vi "delay.vi"(8 "error in":errorcluster, 10 "Milliseconds to wait":i32=50, 11 "VISA resource name":refnum<visa-resource-name>) -> (0 "error out":errorcluster, 3 "VISA resource name out":refnum<visa-resource-name> caption="VISA resource name")   [LabVIEW 2014, in "rszvl_rsidr_core.lvlib"]
uses:
  rszvl_rsidr_core.lvlib
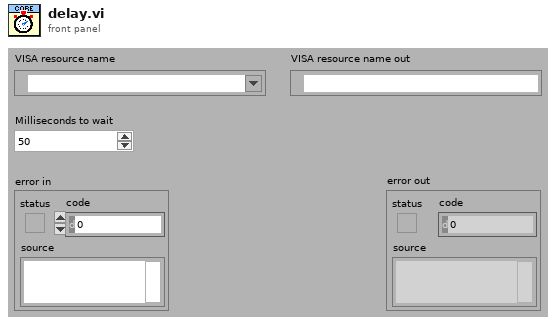
[diagram p1: front panel]
types:
  T1 = typedef "rszvl_rsidr_core.lvlib/type_Session_Data.ctl" = cluster{"Instr type":string, "Instr type for err. msg.":string, "Installed Options":string[], "OPC Timeout":i32, "Query Instrument Status":bool, "Check Range":bool, "Check Options":bool, "Add LF to Write":bool, "Simulate":bool, "Logging":bool, "Logging params":variant, "Interface Type":enum16{"Unknown", "GPIB", "VXI", "GPIB_VXI", "ASRL", "PXI", "TCPIP", "USB", "SOCKET"}, "Fast Sweep":i32, "AdditionalFlags":i32, "WaitBeforeWrite":i32, "WaitBeforeRead":i32, "BinDataChunkSize":i64}
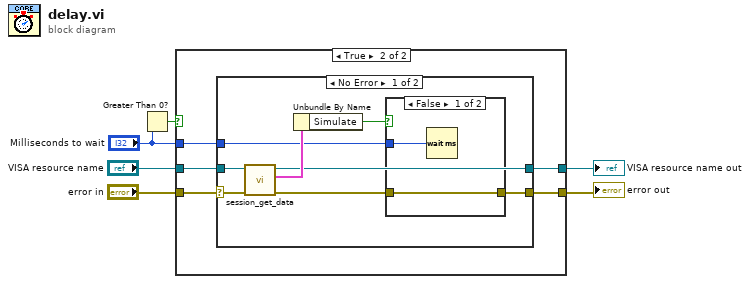
[diagram p0: block diagram]
diagram:
  n1 = Greater Than 0?(x="Milliseconds to wait") -> (x > 0?=w2:bool)
  n2 = case shown="True" w2 {
    tunnel: [w8 w13] -> w6
    tunnel: "VISA resource name" -> [w7 w12]
    tunnel: "error in" -> [w8 w11]
    tunnel: "Milliseconds to wait" -> [_ w10]
    tunnel: [w7 w9] -> w1
    frame False {
    }
    frame True {
      n3 = case shown="No Error" w11 {
        selector: w11 -> [w20 w26]
        tunnel: [w21 w26] -> w13
        tunnel: w12 -> [w19 w25]
        tunnel: w10 -> [w15 _]
        tunnel: [w14 w25] -> w9
        frame No Error {
          n4 = call "session_get_data.vi"("error in"=w20, "VISA resource name"=w19) -> ("error out"=w18:errorcluster, "Session User Data out"=w17:T1, "VISA resource name out"=w14:refnum<visa-resource-name>)  [unwired: 7 in]
          n5 = Unbundle By Name(w17) -> ("Simulate"=w16:bool)
          n6 = case shown="False" w16 {
            tunnel: [w23 w24] -> w21
            tunnel: w18 -> [w23 w24]
            tunnel: w15 -> [w22 _]
            frame False {
              n7 = Wait (ms)(milliseconds to wait=w22) -> ()  [unwired: 1 out]
            }
            frame True {
            }
          }
        }
        frame Error {
        }
      }
    }
  }
  "VISA resource name out" <- w1
  "error out" <- w6
